vi "Get BaseNodeType.vi"(8 "error in":errorcluster, 11 "item in":T1 format="%.0x") -> (0 "error out":errorcluster, 2 "BaseNodeType":refnum<k24>, 3 "item out":T1 format="%.0x")   [LabVIEW 2019, in "Routing and Faulting Scripting.lvlib"]
uses:
  Routing and Faulting Scripting.lvlib
  <vilib>/NI VeriStand/Custom Device API/Custom Device Item Ref.ctl
  NationalInstruments.VeriStand.SystemStorage
  NationalInstruments.VeriStand.SystemDefinitionAPI
  <vilib>/NI VeriStand/Custom Device API/Custom Device API.lvlib
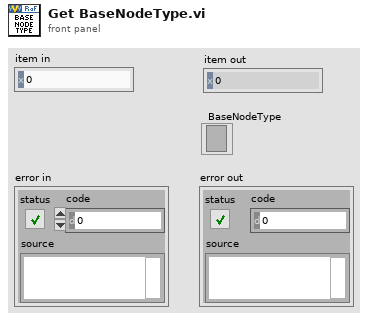
[diagram p1: front panel]
types:
  T1 = typedef "Custom Device API.lvlib/Custom Device Item Ref.ctl" = u64
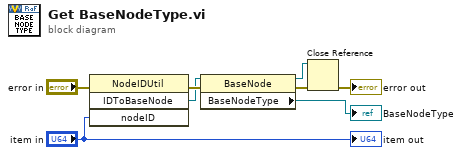
[diagram p0: block diagram]
diagram:
  n1 = invoke class="NodeIDUtil" method="IDToBaseNode"(error in="error in", "nodeID"="item in") -> (error out=w8:errorcluster, "IDToBaseNode"=w7:refnum<k24>)  [unwired: 2 in, 2 out]
  n2 = property class="BaseNode"(reference=w7, error in=w8) -> (reference out=w5:refnum<k24>, error out=w6:errorcluster, "BaseNodeType"=→"BaseNodeType":refnum<k24>)
  n3 = Close Reference(reference=w5, error in (no error)=w6) -> (error out=→"error out":errorcluster)
  "item out" <- "item in"
